vi "Activity_2.vi"() -> ()   [LabVIEW 2015]
panel:
  in  "Stop":bool
  out "Time Stamp 2":timestamp
  in  "Time Stamp":timestamp=timestamp(3632585203.3545537 s since 1904-01-01)
  out "Enum 2":enum16{"Uno", "Dos", "Tres"}(ring)
  in  "Enum":enum16{"Uno", "Dos", "Tres"}(ring)
  out "Ring 4":u16(ring)
  in  "Ring 3":u16(ring) items=["Uno", "Dos"]
  out "Ring 2":u16(ring)
  in  "Ring":u16(ring) items=["Uno", "Dos"]
  out "Cluster 2":T1
  in  "Cluster":T2={"Numeric Control"=8.0, "Switch"=FALSE, "String Capture"="Hellooo"}
  out "Array 4":string[](array[string])=["Hello", "Mine", "Turtle"]
  out "Array 3":dbl[](array[numeric])=[1.0, 2.2, 3.0, 45.06, 0.07]
  in  "Array 2":string[](array[string])=["Hello", "Mine", "Turtle"]
  in  "Array":dbl[](array[numeric])=[1.0, 2.2, 3.0, 45.06, 0.07]
  out "Path Display":path=path "C:/Users/leser/Dropbox/Equipo9/Activity_2.vi"
  in  "Path":path=path "C:/Users/leser/Dropbox/Equipo9/Activity_2.vi"
  out "String Const":string="Hola"
  out "String Display":string="Hello"
  in  "String Capture":string="Hello"
  out "Led":bool
  in  "Switch":bool
  out "Numeric Display":dbl=3.0 format="%.2f"
  out "Numeric Const":dbl=4.0
  in  "Numeric Control":dbl=3.0
  # "Controles e Indicadores"
  # "Fecha de Entrega: 9/2/2019"
  # "Objetivo: Conocer, manipular y cambiar las\npropiedades de los controles e indicadores"
  # "Serrano Bermúdez Luis Esteban"
  # "Programa que controlsa los\ndiferentes tipos de datos de\nLabView"
  # "Descripción:"
  # "Timestamp"
  # "Controls -> Numeric"
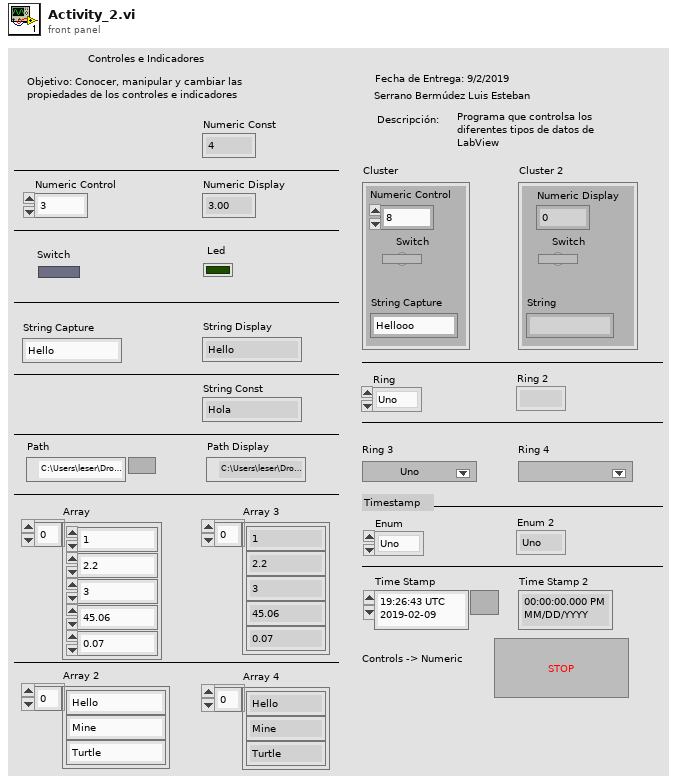
[diagram p1: front panel]
types:
  T1 = cluster{"Numeric Display":dbl, "Switch":bool, "String":string}
  T2 = cluster{"Numeric Control":dbl, "Switch":bool, "String Capture":string}
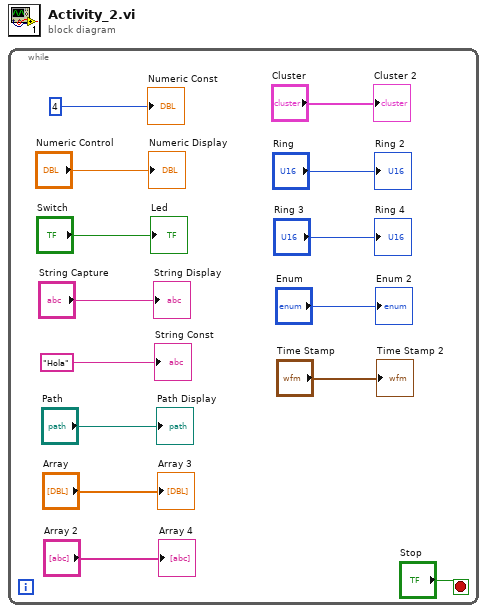
[diagram p0: block diagram]
diagram:
  n1 = while {
    stop <- "Stop" stop-if-true
    "Numeric Const" <- 4
    "Numeric Display" <- "Numeric Control"
    "Led" <- "Switch"
    "String Display" <- "String Capture"
    "String Const" <- "Hola"
    "Path Display" <- "Path"
    "Array 3" <- "Array"
    "Array 4" <- "Array 2"
    "Cluster 2" <- "Cluster"
    "Ring 2" <- "Ring"
    "Ring 4" <- "Ring 3"
    "Enum 2" <- "Enum"
    "Time Stamp 2" <- "Time Stamp"
  }
